vi "project_subject.vi"() -> ()   [LabVIEW 2015]
uses:
  <vilib>/LabVIEW Open Source Project/MQTT Control Packets/Control Packets/SUBACK/Subscription Success Code.ctl
  <vilib>/LabVIEW Open Source Project/MQTT Control Packets/Control Packets/ControlPacket/QualityOfService -- enum.ctl
  <vilib>/LabVIEW Open Source Project/MQTT Control Packets/Control Packets/SUBSCRIBE/Topic Subscription -- cluster.ctl
  <vilib>/LabVIEW Open Source Project/MQTT Control Packets/Control Packets/CONNECT/ConnectFlags -- cluster.ctl
  <vilib>/LabVIEW Open Source Project/MQTT Client/Client class/Client.lvclass/Client.ctl
  <vilib>/LabVIEW Open Source Project/MQTT Connection/MQTT_Base/Base Class/MQTT_Base.lvclass/MQTT_Base.ctl
  <vilib>/LabVIEW Open Source Project/MQTT Control Packets/Control Packets/ControlPacket/ControlPacket.lvclass/ControlPacket.ctl
  <vilib>/Modbus/master/Create Master Instance (Serial).vi
  <vilib>/LabVIEW Open Source Project/MQTT Control Packets/Control Packets/PUBLISH/PUBLISH.lvclass
  <vilib>/Modbus/master/Modbus Master.lvclass
  <vilib>/LabVIEW Open Source Project/MQTT Client/Client class/Client.lvclass
  <vilib>/LabVIEW Open Source Project/MQTT Connection/MQTT_Base/Base Class/MQTT_Base.lvclass
  <vilib>/LabVIEW Open Source Project/MQTT Control Packets/Control Packets/ControlPacket/ControlPacket.lvclass
  <vilib>/LabVIEW Open Source Project/Connection/Connection.TCP/Connection.TCP.lvclass
  <vilib>/LabVIEW Open Source Project/Connection/Connection.LocalQueue/Connection.LocalQueue.lvclass
  <vilib>/LabVIEW Open Source Project/Connection/Connection/Connection.lvclass
  <vilib>/LabVIEW Open Source Project/MQTT Control Packets/Control Packets/SUBACK/SUBACK.lvclass
  <vilib>/LabVIEW Open Source Project/MQTT Control Packets/Control Packets/SUBSCRIBE/SUBSCRIBE.lvclass
  <vilib>/LabVIEW Open Source Project/MQTT Control Packets/Control Packets/CONNECT/CONNECT.lvclass
panel:
  out "source 2":string
  out "code":i32
  out "status":bool
  out "source":string
  in  "stop 2":bool
  out "concatenated string":string
  in  "error in (no error)":errorcluster
  in  "ID (empty:generate new)":string="3822e249-e744-453b-bbf7-de2d9c82744f"
  in  "Connect Flags":T1={"Reserved"=FALSE, "Clean Session"=TRUE, "Will Flag"=FALSE, "Will QoS 1"=FALSE, "Will QoS 2"=FALSE, "Will Retain"=FALSE, "Password Flag"=TRUE, "User Name Flag"=TRUE}
  out "error out 7":errorcluster
  in  "Payload":T2={"Will Topic"="", "Will Message"="", "Username"="FqAEnQLp1Sw4eE9xSTHCFsPptqUtCBk6", "Password"="ruWF9yMR2DR78Q5ppRGFwd8ujJNSitBF"}
  out "error out 2":errorcluster
  out "Incoming Message":u8[](array[numeric]) format="%08b"
  out "error out 6":errorcluster
  out "Data2":string
  out "Type 2":variant
  out "Topic 2":string
  out "error out 5":cluster{}
  out "error out 4":errorcluster
  out "Data1":string
  out "Type":variant
  out "Topic":string
  out "error out 3":cluster{"status":bool, "code":i32}
  in  "Subscribe":bool
  in  "Topic Subscriptions":T3[](array[typedef])=[{"Topic Filter"="@msg/D1/LED1", "QoS"=enum."0 (At Most Once)"}]
  out "Subscription Success":T5[](array[typedef])
  out "Suback":bool
  out "Published":bool
  out "number (0 to 1)":dbl
  in  "Publish":bool
  in  "Stop Client":bool
  in  "SET POINT":dbl
  out "Huminity":dbl(knob) scale=0.0..100.0
  out "Numeric":i32
  out "element":u16
  out "Gauge":dbl(knob) scale=0.0..500.0
  in  "Knob Set Speed":i32(knob) scale=0.0..100.0
  in  "address":u16=100
  in  "holding register value":u16
  in  "Write Button":bool
  in  "baud rate (9600)":u32=9600
  in  "flow control (None)":u16(ring) items=["None", "XON/XOFF", "RTS/CTS", "XON/XOFF & RTS/CTS", "DTR/DSR", "XON/XOFF & DTR/DSR"]
  in  "parity (Even)":u16(ring) items=["None", "Odd", "Even"]
  in  "unit ID":u8=10
  out "error out":errorcluster
  out "register values":u16[](array[numeric])
  in  "number of input registers":u16=10
  in  "starting address":u16=100
  in  "stop":bool
  in  "serial type":enum16{"RTU", "ASCII"}(ring)
  in  "VISA resource name":refnum<visa-resource-name>
  # "The light turns on when the water is turned on."
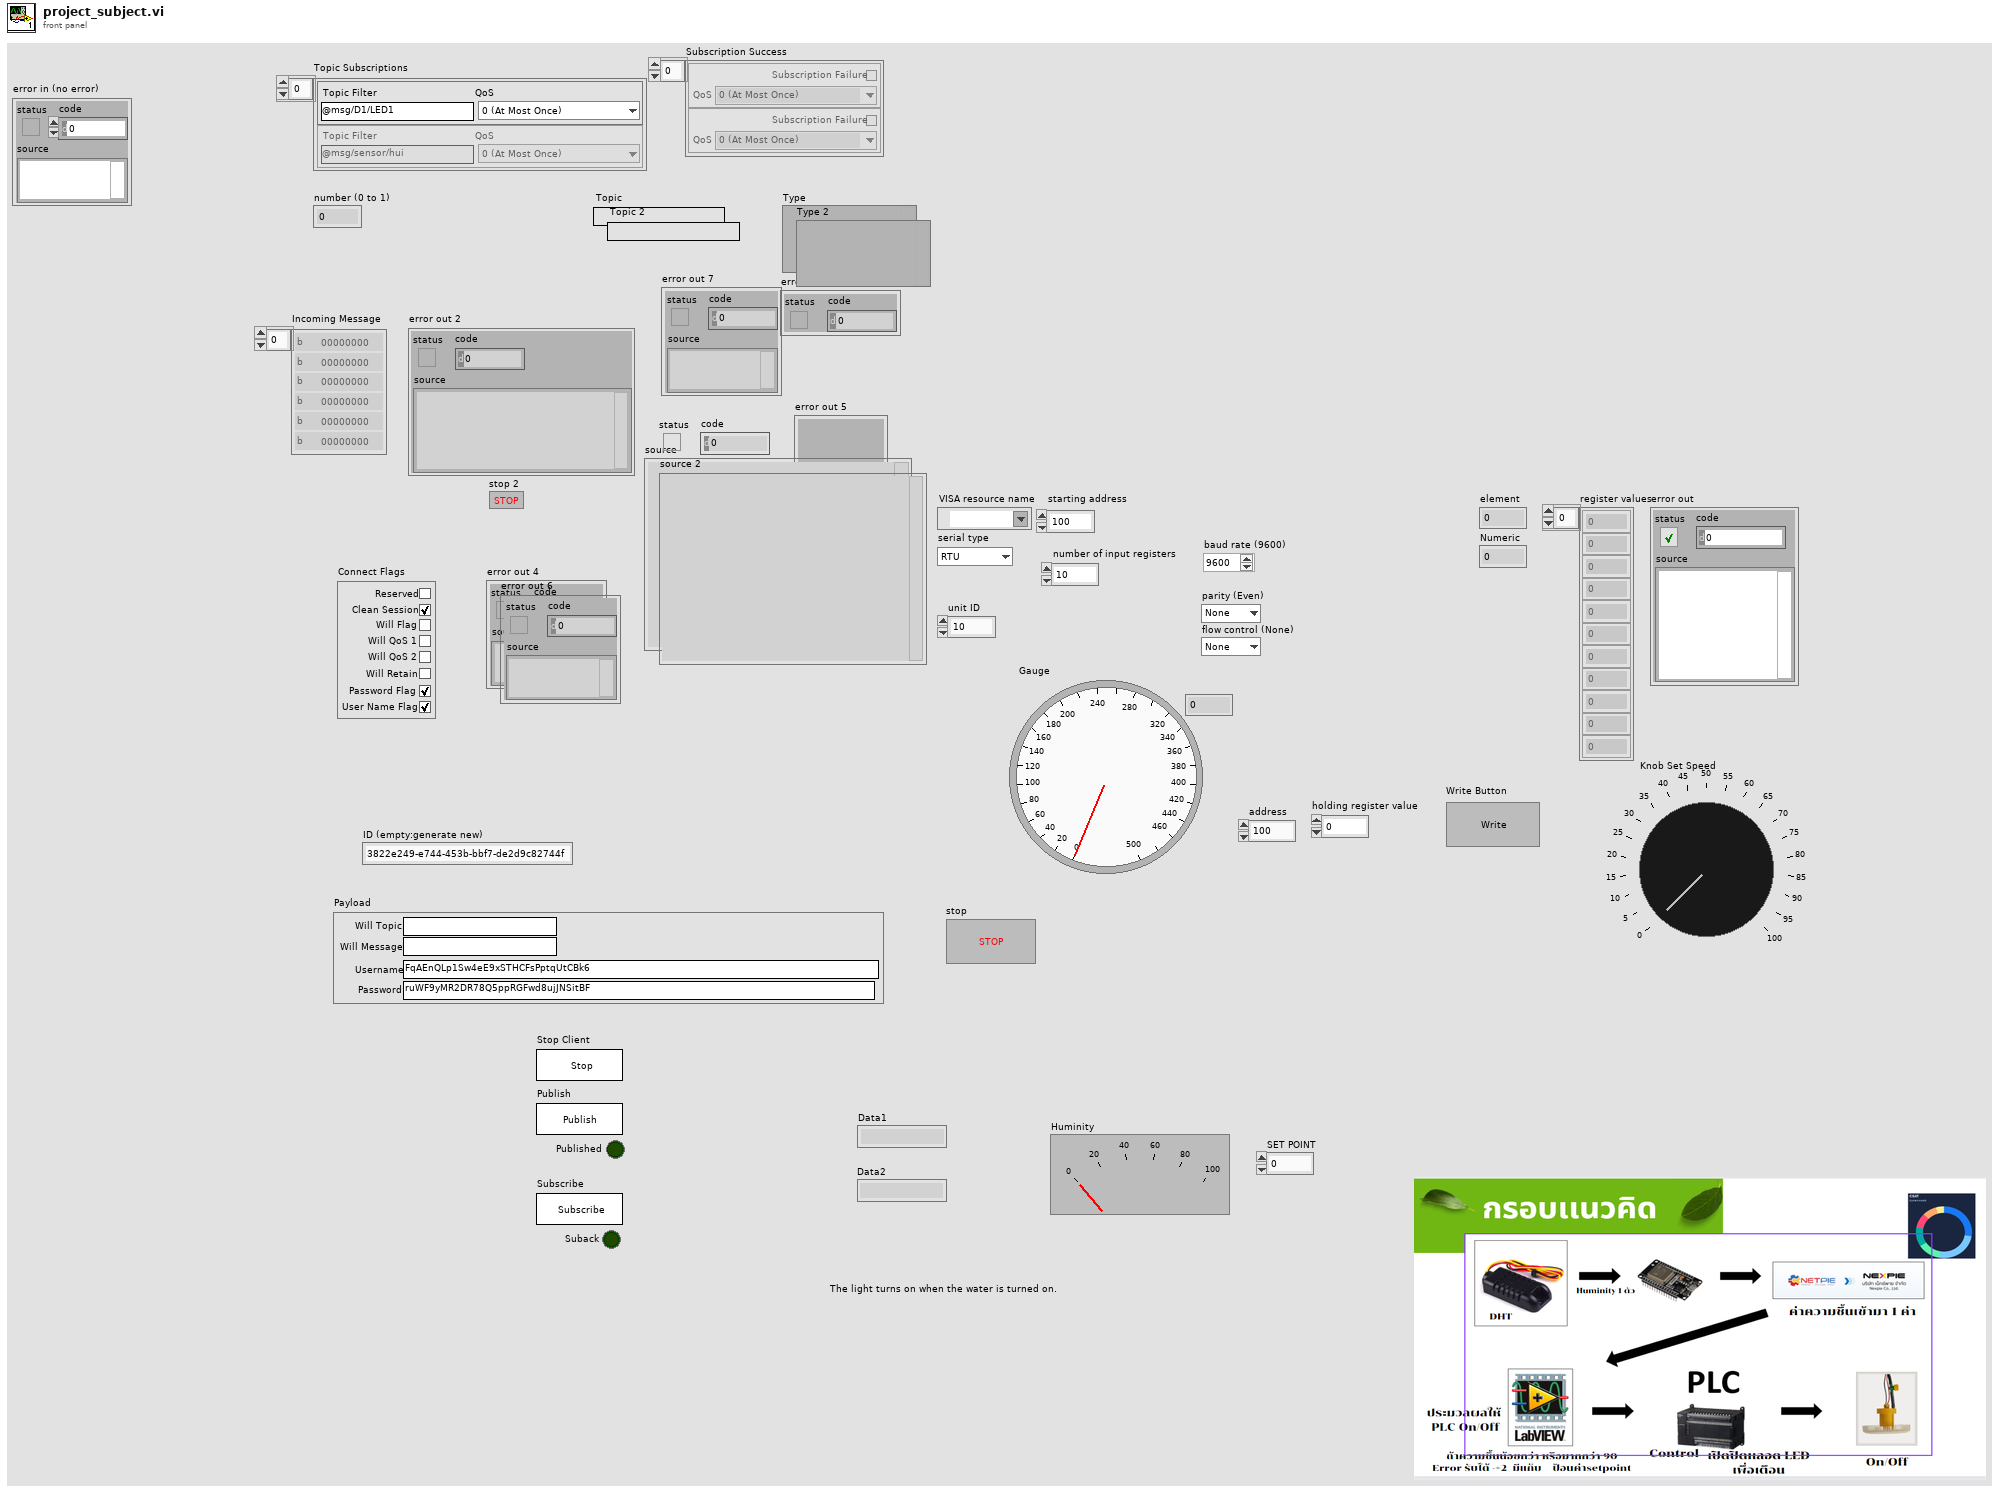
[diagram p1: front panel]
types:
  T1 = typedef "MQTT_Control_Packets.lvlib/CONNECT.lvclass/ConnectFlags -- cluster.ctl" = cluster{"Reserved":bool, "Clean Session":bool, "Will Flag":bool, "Will QoS 1":bool, "Will QoS 2":bool, "Will Retain":bool, "Password Flag":bool, "User Name Flag":bool}
  T2 = cluster{"Will Topic":string, "Will Message":string, "Username":string, "Password":string}
  T3 = typedef "MQTT_Control_Packets.lvlib/SUBSCRIBE.lvclass/Topic Subscription -- cluster.ctl" = cluster{"Topic Filter":string, "QoS":T4}
  T4 = typedef "MQTT_Control_Packets.lvlib/ControlPacket.lvclass/QualityOfService -- enum.ctl" = enum16{"0 (At Most Once)", "1 (At Least Once)", "2 (Exactly Once)"}
  T5 = typedef "MQTT_Control_Packets.lvlib/SUBACK.lvclass/Subscription Success Code.ctl" = cluster{"Subscription Failure":bool, "QoS":T4}
  T6 = typedef "MQTT Client.lvlib/Client.lvclass/Public Events -- cluster.ctl" = cluster{"Connection Status":refnum<user-event>, "Connected":refnum<user-event>, "Application Message":refnum<user-event>}
  T7 = typedef "MQTT Base.lvlib/MQTT_Base.lvclass/Public Events -- cluster.ctl" = cluster{"Stop Event":refnum<user-event>, "Error Event":refnum<user-event>, "Inbound Message":refnum<user-event>}
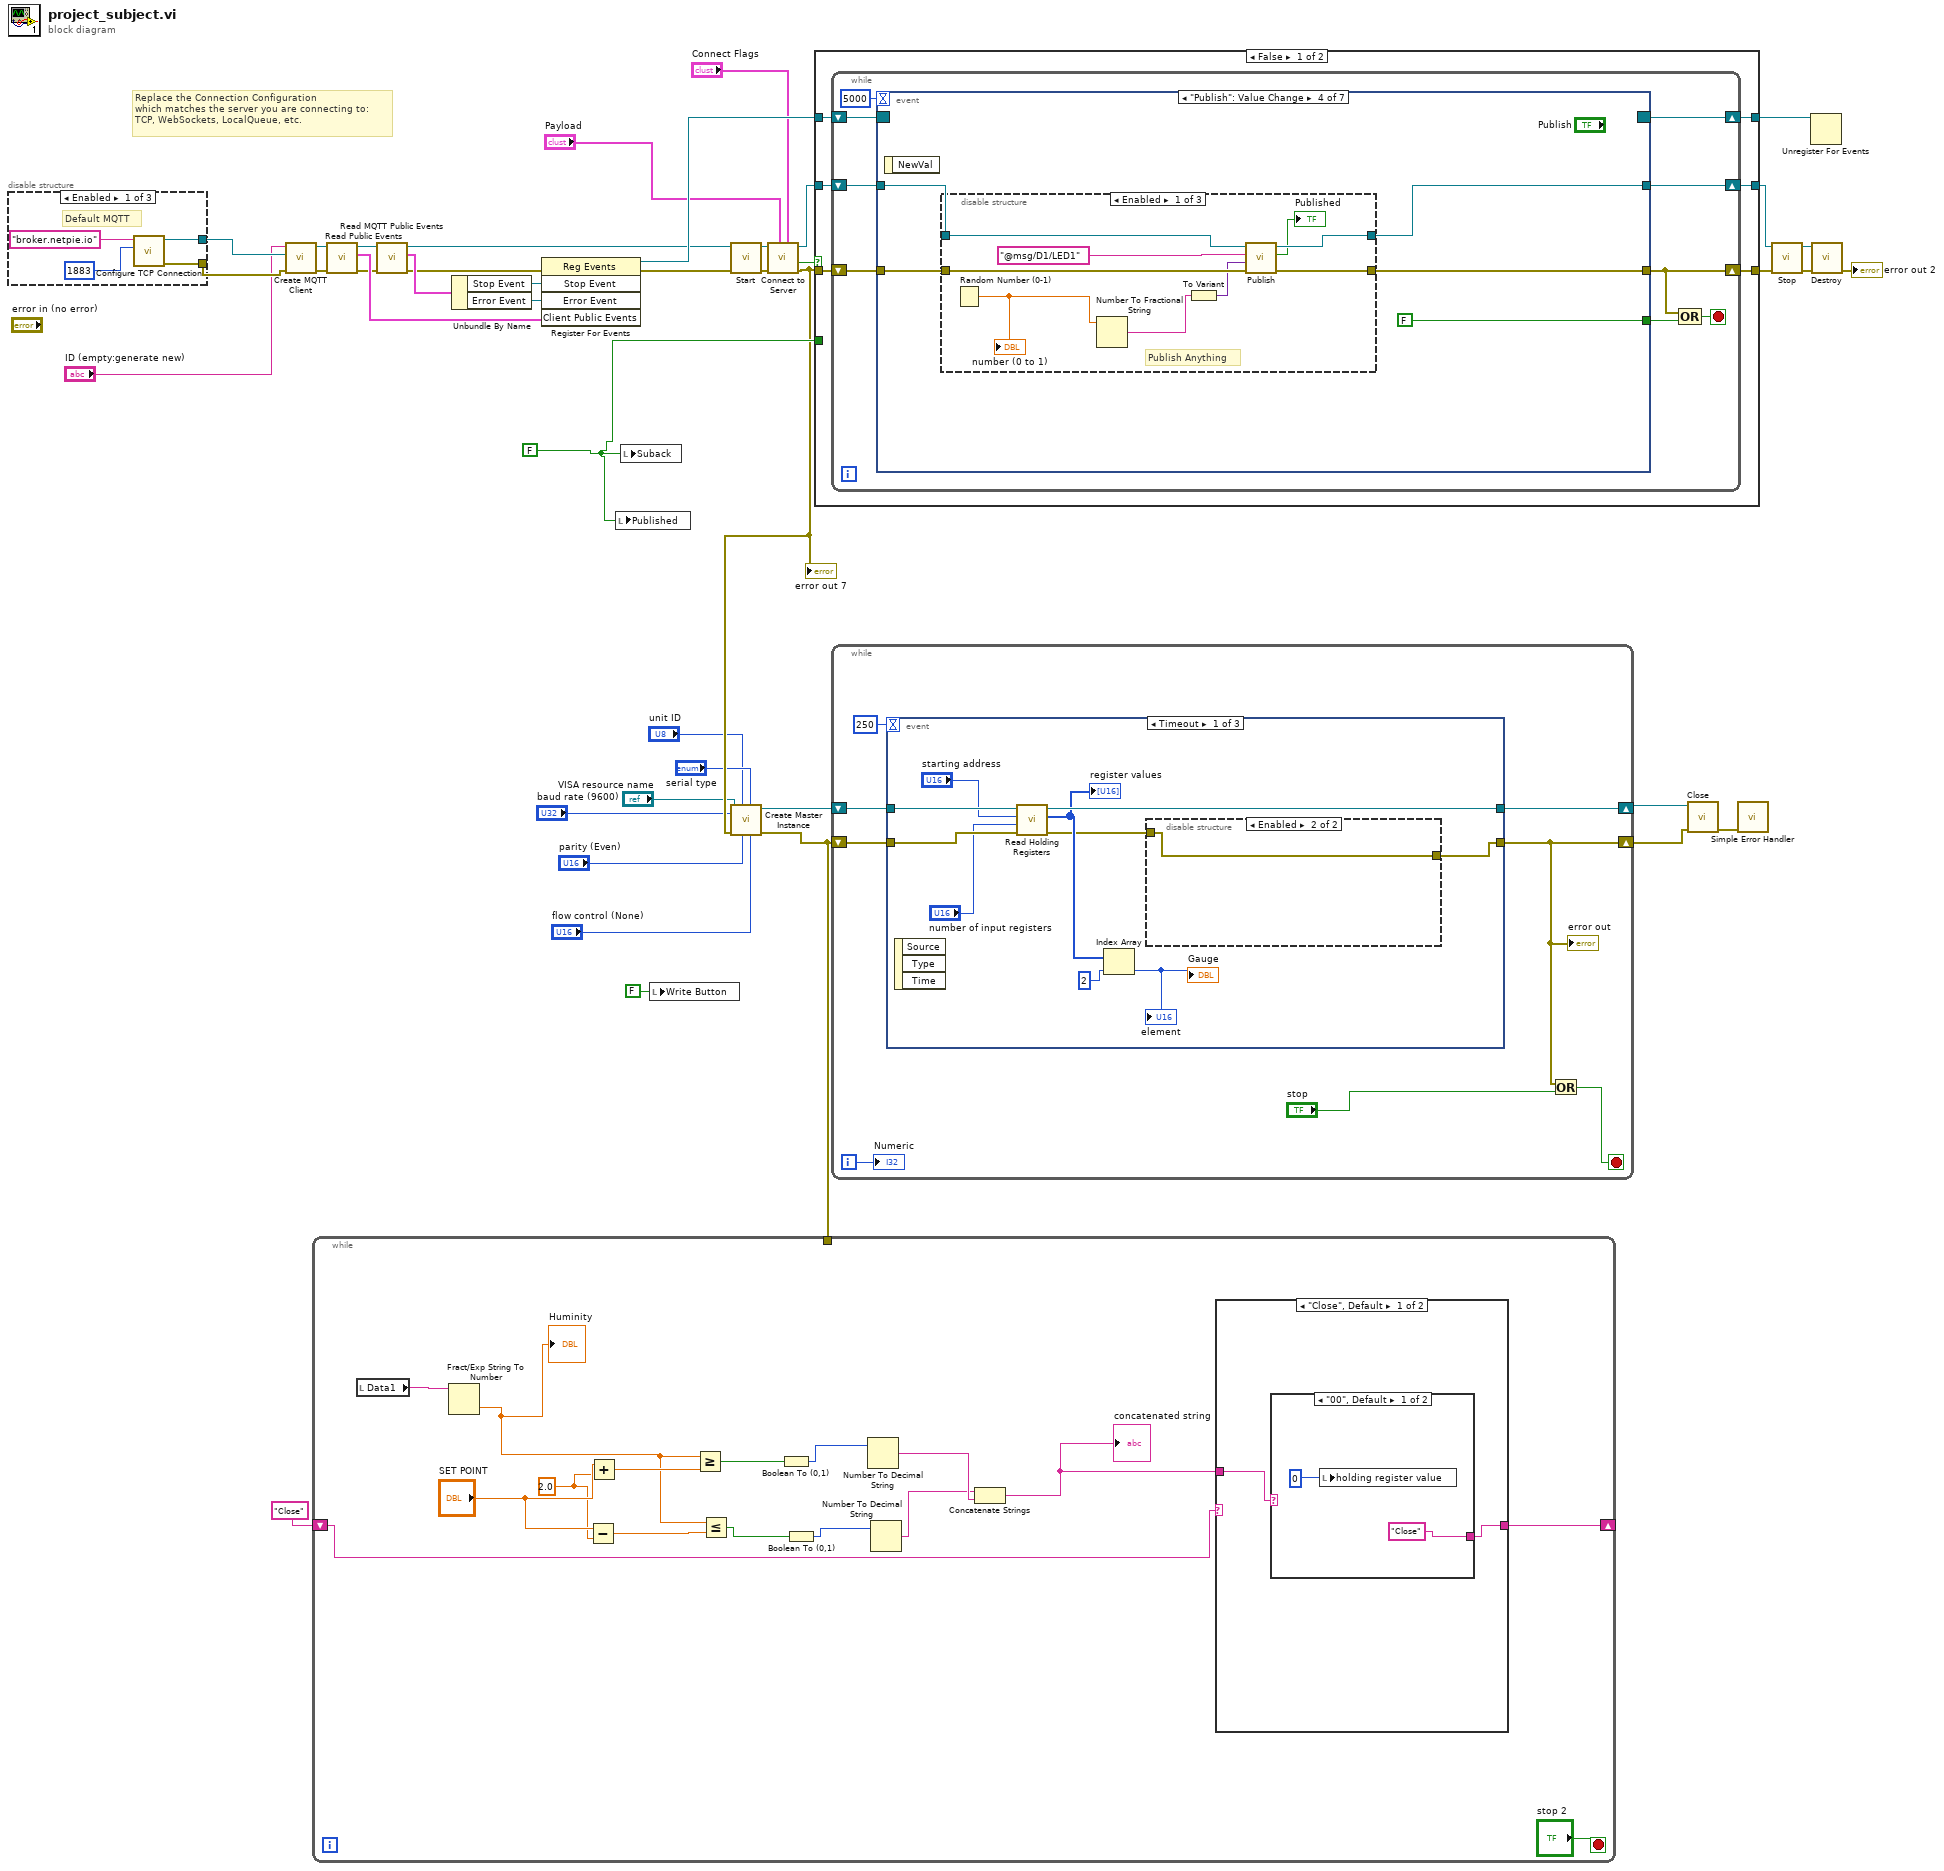
[diagram p0: block diagram]
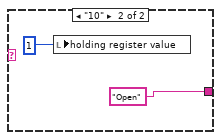
[diagram p2: hidden frame]
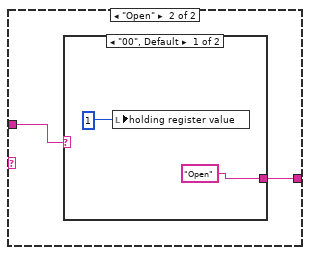
[diagram p3: hidden frame]
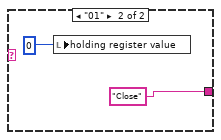
[diagram p4: hidden frame]
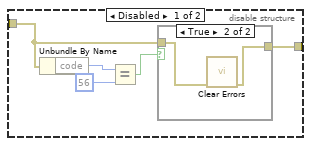
[diagram p5: hidden frame]
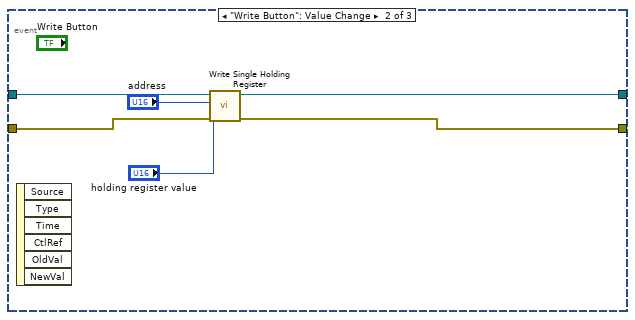
[diagram p7: hidden frame]
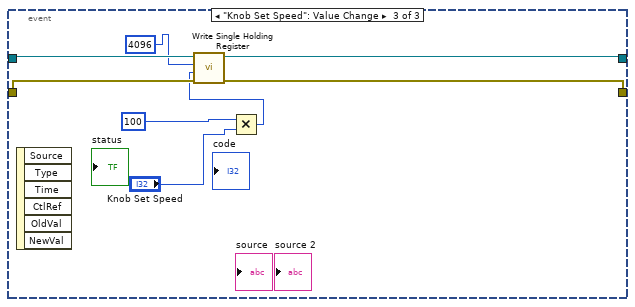
[diagram p8: hidden frame]
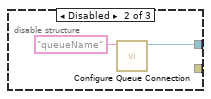
[diagram p9: hidden frame]
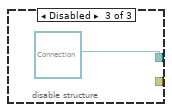
[diagram p10: hidden frame]
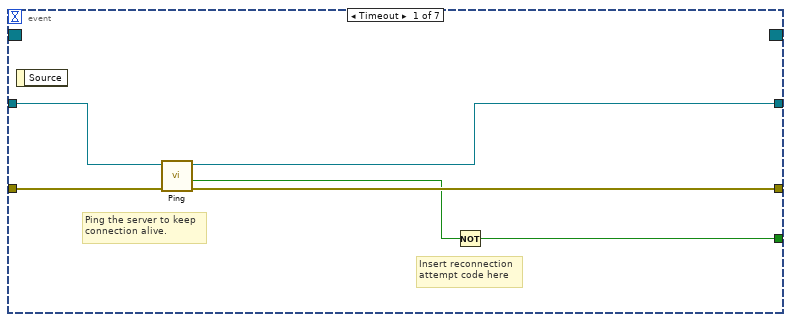
[diagram p11: hidden frame]
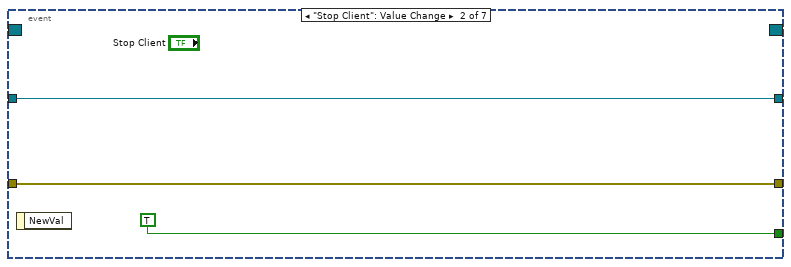
[diagram p12: hidden frame]
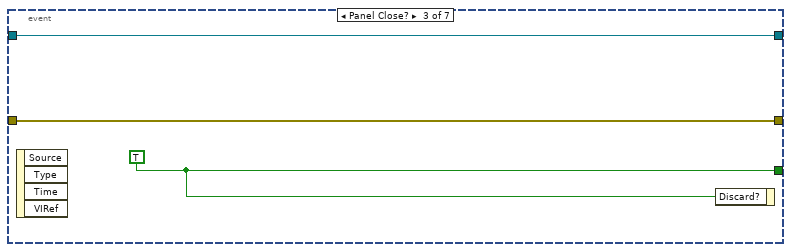
[diagram p13: hidden frame]
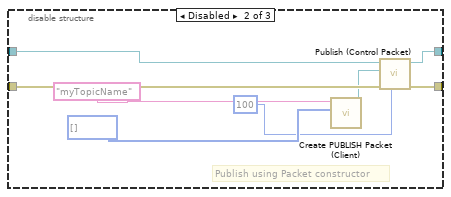
[diagram p14: hidden frame]
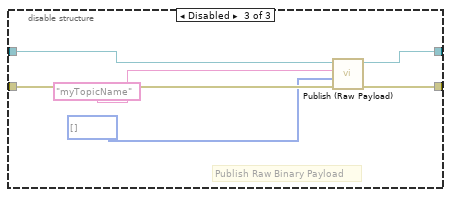
[diagram p15: hidden frame]
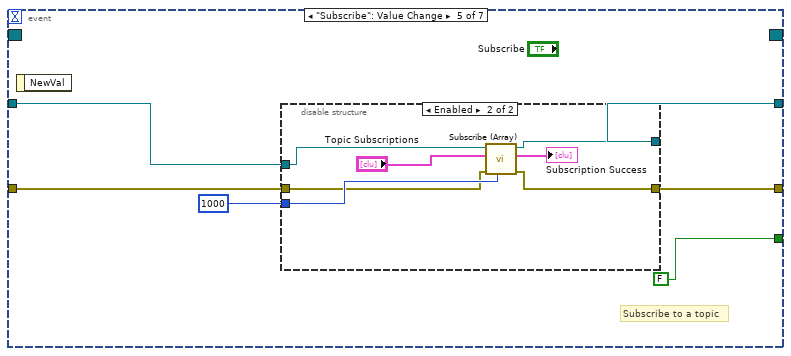
[diagram p16: hidden frame]
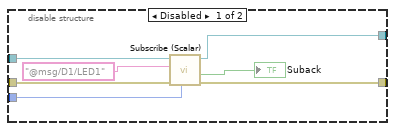
[diagram p17: hidden frame]
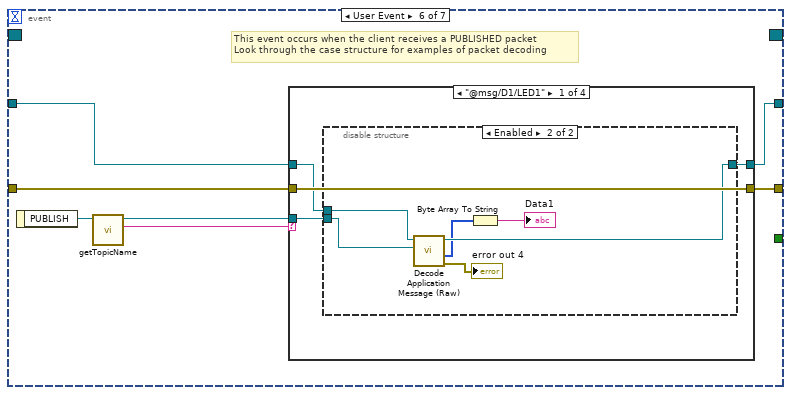
[diagram p18: hidden frame]
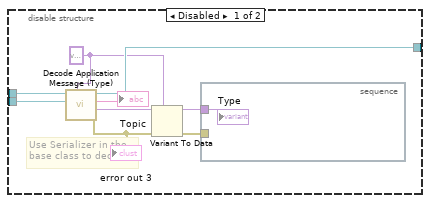
[diagram p19: hidden frame]
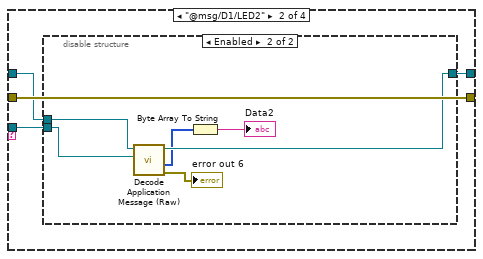
[diagram p20: hidden frame]
diagram:
  w16 = FALSE ("Suback")
  # "Replace the Connection Configuration\nwhich matches the server you are connecting to:\nTCP, WebSockets, LocalQueue, etc."
  n1 = disable-structure shown="Enabled" {
    disable-tunnel: [w45 w48 refnum<class "Connection.lvclass"> refnum ("Connection Configuration")] -> w42
    disable-tunnel: [w43 _ _] -> w19
    frame Enabled {
      # "Default MQTT"
      n2 = call <vilib>:"Configure TCP Connection.vi"("remote port (80)"=u16 1883, "address (localhost)"="broker.netpie.io") -> ("error out"=w43:errorcluster, "Connection.TCP"=w45:refnum<class "Connection.TCP.lvclass">)  [unwired: 8 in]
    }
    frame Disabled {
      n3 = call <vilib>:"Configure Queue Connection.vi"("Queue Name"="queueName") -> ("Connection.LocalQueue"=w48:refnum<class "Connection.LocalQueue.lvclass">)  [unwired: 9 in, 1 out]
    }
    frame Disabled {
    }
  }
  n4 = call <vilib>:"Create MQTT Client.vi"("error in (no error)"=w19, "Connection Configuration"=w42, "ID (empty:generate new)"="ID (empty:generate new)") -> ("error out"=w22:errorcluster, "Client out"=w20:refnum<class "Client.lvclass">)  [unwired: 7 in]
  n5 = call <vilib>:"Read Public Events.vi"("error in (no error)"=w22, "Client in"=w20) -> ("error out"=w23:errorcluster, "Client Public Events"=w25:T6, "Client out"=w21:refnum<class "Client.lvclass">)  [unwired: 7 in]
  n6 = call <vilib>:"Read MQTT Public Events.vi"("error in (no error)"=w23, "MQTT_Base in"=w21) -> ("error out"=w24:errorcluster, "MQTT Public Events"=w36:T7, "MQTT_Base out"=w27:refnum<class "Client.lvclass">)  [unwired: 7 in]
  n7 = Unbundle By Name(w36) -> ("Stop Event"=w34:refnum<user-event>, "Error Event"=w35:refnum<user-event>)
  n8 = register-events(error in=w24, w34, w35, w25) -> (reference out=w30:refnum<event-registration>, error out=w26:errorcluster)  [unwired: 1 in]
  n9 = local write "Published"(w16) -> ()
  n10 = local write "Suback"(w16) -> ()
  n11 = local write "Write Button"(FALSE ("Write Button")) -> ()
  n12 = call <vilib>:"Start.vi"("error in (no error)"=w26, "MQTT_Base in"=w27) -> ("error out"=w29:errorcluster, "MQTT_Base out"=w28:refnum<class "Client.lvclass">)  [unwired: 7 in, 1 out]
  n13 = call <vilib>:"Connect to Server.vi"("Connect Flags"="Connect Flags", "Payload"="Payload", "error in (no error)"=w29, "Client in"=w28) -> ("error out"=w15:errorcluster, "timed out"=w32:bool, "Client out"=w33:refnum<class "Client.lvclass">)  [unwired: 4 in, 1 out]
  "error out 7" <- w15
  n14 = call-poly <vilib>:"Create Master Instance.vi"("flow control (None)"="flow control (None)", "serial type"="serial type", "parity (Even)"="parity (Even)", "unit ID"="unit ID", "error in (no error)"=w15, "baud rate (9600)"="baud rate (9600)", "VISA resource name"="VISA resource name") -> ("error out"=w2:errorcluster, "serial master instance"=w11:refnum<class "Modbus Master.lvclass">)  [unwired: 3 in]
  n15 = while {
    tunnel: w2 -> [_]
    shift-right: [w52] -> _
    shift-left: "Close" -> [w53]
    stop <- "stop 2" stop-if-true
    w63 = 2.0 ("y")
    n16 = local read "Data1"() -> (w65:string)
    n17 = Fract/Exp String To Number(string=w65) -> (number=w50:dbl)  [unwired: 3 in, 1 out]
    "Huminity" <- w50
    n18 = Subtract(x="SET POINT", y=w63) -> (x-y=w61:dbl)
    n19 = Add(x="SET POINT", y=w63) -> (x+y=w62:dbl)
    n20 = Greater Or Equal?(x=w50, y=w62) -> (x >= y?=w60:bool)
    n21 = Less Or Equal?(x=w50, y=w61) -> (x <= y?=w59:bool)
    n22 = Boolean To (0,1)(Boolean=w60) -> (0, 1=w58:i16)
    n23 = Boolean To (0,1)(Boolean=w59) -> (0, 1=w57:i16)
    n24 = Number To Decimal String(number=w58) -> (decimal integer string=w56:string)  [unwired: 1 in]
    n25 = Number To Decimal String(number=w57) -> (decimal integer string=w55:string)  [unwired: 1 in]
    n26 = Concatenate Strings(w55, w56) -> (w54:string)
    "concatenated string" <- w54
    n27 = case shown="\"Close\", Default" w53 {
      tunnel: w54 -> [w66 w73]
      tunnel: [w67 w72] -> w52
      frame "Close", Default {
        n28 = case shown="\"00\", Default" w66 {
          tunnel: ["Close" "Open"] -> w67
          frame "00", Default {
            n29 = local write "holding register value"(u16 0 ("holding register value")) -> ()
          }
          frame "10" {
            n30 = local write "holding register value"(u16 1 ("holding register value")) -> ()
          }
        }
      }
      frame "Open" {
        n31 = case shown="\"00\", Default" w73 {
          tunnel: ["Open" "Close"] -> w72
          frame "00", Default {
            n32 = local write "holding register value"(u16 1 ("holding register value")) -> ()
          }
          frame "01" {
            n33 = local write "holding register value"(u16 0 ("holding register value")) -> ()
          }
        }
      }
    }
  }
  n34 = case shown="False" w32 {
    tunnel: w30 -> [w83 w215]
    tunnel: [w82 w215] -> w31
    tunnel: w15 -> [w79 w213]
    tunnel: w33 -> [w81 w214]
    tunnel: [w80 w214] -> w38
    tunnel: [w78 w213] -> w40
    tunnel: w16 -> [_ _]
    frame False {
      n35 = while {
        shift-right: [w91] -> w82
        shift-left: w83 -> [w92]
        shift-right: [w84] -> w80
        shift-left: w81 -> [w85]
        shift-right: [w89] -> w78
        shift-left: w79 -> [w90]
        stop <- w88 stop-if-true
        n36 = event shown="[3] \"Publish\": Value Change" {
          selector: w92 -> [_ _ _ _ _ _ _]
          dyn-events: [_ _ _ _ _ _ _] -> w91
          timeout: 5000 -> [_ _ _ _ _ _ _]
          tunnel: w90 -> [w97 w100 w102 w107 w136 w154 w212]
          tunnel: [w95 w100 w102 w106 w135 w155 w212] -> w89
          tunnel: [w94 TRUE w104 FALSE FALSE _ TRUE] -> w87
          tunnel: w85 -> [w98 w101 w103 w108 w137 w157 w210]
          tunnel: [w96 w101 w103 w105 w134 w156 w210] -> w84
          event Timeout {
            # "Insert reconnection\nattempt code here"
            # "Ping the server to keep\nconnection alive."
            n37 = event-data() -> ()  [unwired: 1 in, 1 out]
            n38 = call <vilib>:"Ping.vi"("error in (no error)"=w97, "Client in"=w98) -> ("error out"=w95:errorcluster, "Server responded"=w93:bool, "Client out"=w96:refnum<class "Client.lvclass">)  [unwired: 6 in, 1 out]
            n39 = Not(x=w93) -> (.not. x?=w94:bool)
          }
          event "Stop Client": Value Change {
            n40 = event-data() -> ()  [unwired: 1 in, 1 out]
          }
          event Panel Close? {
            w104 = TRUE
            n41 = event-data() -> ()  [unwired: 1 in, 4 out]
            n42 = event-data("Discard?"=w104) -> ()  [unwired: 1 in, 1 out]
          }
          event "Publish": Value Change {
            n43 = event-data() -> ()  [unwired: 1 in, 1 out]
            n44 = disable-structure shown="Enabled" {
              disable-tunnel: w108 -> [w118 w124 w132]
              disable-tunnel: w107 -> [w117 w122 w129]
              disable-tunnel: [w116 w121 w130] -> w106
              disable-tunnel: [w115 w123 w131] -> w105
              frame Enabled {
                # "Publish Anything"
                n45 = Random Number (0-1)() -> (number: 0 to 1=w111:dbl)
                "number (0 to 1)" <- w111
                n46 = Number To Fractional String(number=w111) -> (F-format string=w110:string)  [unwired: 3 in]
                n47 = To Variant(anything=w110) -> (Variant=w113:variant)
                n48 = call <vilib>:"Publish.vi"("error in (no error)"=w117, "Payload"=w113, "Topic Name (empty: Payload name)"="@msg/D1/LED1", "Client in"=w118) -> ("error out"=w116:errorcluster, "Published"=→"Published":bool, "Client out"=w115:refnum<class "Client.lvclass">)  [unwired: 5 in]
              }
              frame Disabled {
                # "Publish using Packet constructor"
                n49 = call <vilib>:"Create PUBLISH Packet (Client).vi"("Payload"=u8[] [], "Topic Name"="myTopicName" ("Topic Name (empty: Payload name)")) -> ("PUBLISH"=w119:refnum<class "PUBLISH.lvclass">)  [unwired: 6 in, 3 out]
                n50 = call <vilib>:"Publish (Control Packet).vi"("timeout (1000ms)"=100 ("timeout (0ms : no ack)"), "error in (no error)"=w122, "PUBLISH"=w119, "Client in"=w124) -> ("error out"=w121:errorcluster, "Client out"=w123:refnum<class "Client.lvclass">)  [unwired: 5 in, 1 out]
              }
              frame Disabled {
                # "Publish Raw Binary Payload"
                n51 = call <vilib>:"Publish (Raw Payload).vi"("error in (no error)"=w129, "Binary Payload"=u8[] [] ("Payload"), "Topic Name"="myTopicName" ("Topic Name (empty: Payload name)"), "Client in"=w132) -> ("error out"=w130:errorcluster, "Client out"=w131:refnum<class "Client.lvclass">)  [unwired: 5 in, 1 out]
              }
            }
          }
          event "Subscribe": Value Change {
            # "Subscribe to a topic"
            n52 = event-data() -> ()  [unwired: 1 in, 1 out]
            n53 = disable-structure shown="Enabled" {
              disable-tunnel: w137 -> [w145 w152]
              disable-tunnel: w136 -> [w143 w148]
              disable-tunnel: [w142 w147] -> w135
              disable-tunnel: [w141 w149] -> w134
              disable-tunnel: 1000 ("timeout (100ms)") -> [w139 w151]
              frame Disabled {
                n54 = call <vilib>:"Subscribe (Scalar).vi"("timeout (1000ms)"=w139, "error in (no error)"=w143, "Topic Filter"="@msg/D1/LED1" ("Topic Name (empty: Payload name)"), "Client in"=w145) -> ("error out"=w142:errorcluster, "Ack"=→"Suback":bool, "Client out"=w141:refnum<class "Client.lvclass">)  [unwired: 5 in]
              }
              frame Enabled {
                n55 = call <vilib>:"Subscribe (Array).vi"("timeout (1000ms)"=w151, "error in (no error)"=w148, "Topic Subscriptions"="Topic Subscriptions", "Client in"=w152) -> ("error out"=w147:errorcluster, "Subscription Success"=→"Subscription Success":T5[], "Client out"=w149:refnum<class "Client.lvclass">)  [unwired: 5 in]
              }
            }
          }
          event User Event {
            # "This event occurs when the client receives a PUBLISHED packet\nLook through the case structure for examples of packet decoding"
            n56 = event-data() -> ("PUBLISH"=w159:refnum<class "PUBLISH.lvclass">)  [unwired: 1 in]
            n57 = call <vilib>:"getTopicName.vi"("PUBLISH in"=w159) -> ("Topic"=w158:string, "PUBLISH out"=w153:refnum<class "PUBLISH.lvclass">)  [unwired: 8 in, 1 out]
            n58 = case shown="\"@msg/D1/LED1\"" w158 {
              tunnel: w157 -> [w162 w182 w205 w209]
              tunnel: [w161 w181 w204 w209] -> w156
              tunnel: [w163 w183 w202 w208] -> w155
              tunnel: w154 -> [w163 w183 w201 w208]
              tunnel: w153 -> [w160 w180 w200 w207]
              frame "@msg/D1/LED1" {
                n59 = disable-structure shown="Enabled" {
                  disable-tunnel: w162 -> [w170 w179]
                  disable-tunnel: [w169 w177] -> w161
                  disable-tunnel: w160 -> [w168 w178]
                  frame Disabled {
                    w166 = variant ("Type")
                    # "Use Serializer in the\nbase class to decode"
                    n60 = call <vilib>:"Decode Application Message (Type).vi"("Type"=w166, "PUBLISH"=w168, "Client in"=w170) -> ("error out"=w165:errorcluster, "Payload"=w167:variant, "Topic"=→"Topic":string, "Client out"=w169:refnum<class "Client.lvclass">)  [unwired: 5 in]
                    "error out 3" <- w165
                    n61 = Variant To Data(error in=w165, type=w166, Variant=w167) -> (data=w172:variant, error out=w171:errorcluster)
                    n62 = stacked-sequence {
                      tunnel: w172 -> [w173]
                      tunnel: w171 -> [_]
                      frame #0 {
                        "Type" <- w173
                      }
                    }
                  }
                  frame Enabled {
                    n63 = call <vilib>:"Decode Application Message (Raw).vi"("PUBLISH"=w178, "Client in"=w179) -> ("error out"=→"error out 4":errorcluster, "Payload"=w175:u8[], "Client out"=w177:refnum<class "Client.lvclass">)  [unwired: 6 in, 1 out]
                    n64 = Byte Array To String(unsigned byte array=w175) -> (string=→"Data1":string)
                  }
                }
              }
              frame "@msg/D1/LED2" {
                n65 = disable-structure shown="Enabled" {
                  disable-tunnel: w182 -> [w190 w199]
                  disable-tunnel: [w189 w197] -> w181
                  disable-tunnel: w180 -> [w188 w198]
                  frame Disabled {
                    w186 = variant ("Type")
                    # "Use Serializer in the\nbase class to decode"
                    n66 = call <vilib>:"Decode Application Message (Type).vi"("Type"=w186, "PUBLISH"=w188, "Client in"=w190) -> ("error out"=w185:errorcluster, "Payload"=w187:variant, "Topic"=→"Topic 2":string, "Client out"=w189:refnum<class "Client.lvclass">)  [unwired: 5 in]
                    "error out 5" <- w185
                    n67 = Variant To Data(error in=w185, type=w186, Variant=w187) -> (data=w192:variant, error out=w191:errorcluster)
                    n68 = stacked-sequence {
                      tunnel: w192 -> [w193]
                      tunnel: w191 -> [_]
                      frame #0 {
                        "Type 2" <- w193
                      }
                    }
                  }
                  frame Enabled {
                    n69 = call <vilib>:"Decode Application Message (Raw).vi"("PUBLISH"=w198, "Client in"=w199) -> ("error out"=→"error out 6":errorcluster, "Payload"=w195:u8[], "Client out"=w197:refnum<class "Client.lvclass">)  [unwired: 6 in, 1 out]
                    n70 = Byte Array To String(unsigned byte array=w195) -> (string=→"Data2":string)
                  }
                }
              }
              frame "RawPayload" {
                n71 = call <vilib>:"Decode Application Message (Raw).vi"("error in (no error)"=w201, "PUBLISH"=w200, "Client in"=w205) -> ("error out"=w202:errorcluster, "Payload"=w203:u8[], "Client out"=w204:refnum<class "Client.lvclass">)  [unwired: 5 in, 1 out]
                n72 = stacked-sequence {
                  tunnel: w203 -> [_]
                  frame #0 {
                  }
                }
              }
              frame Default {
                # "Read Raw Payload"
                n73 = call <vilib>:"Read Payload.vi"("ControlPacket in"=w207) -> ("Payload"=→"Incoming Message":u8[])  [unwired: 9 in, 1 out]
              }
            }
          }
          event User Event {
            n74 = event-data() -> ()  [unwired: 1 in, 1 out]
          }
        }
        n75 = Compound Arithmetic op=OR(w89, w87) -> (w88:bool)
      }
    }
    frame True {
    }
  }
  n76 = while {
    shift-right: [w220] -> w8
    shift-left: w11 -> [w223]
    shift-right: [w219] -> w9
    shift-left: w2 -> [w222]
    i -> [w216]
    stop <- w221 stop-if-true
    n77 = event shown="[0] Timeout" {
      selector: _ -> [_ _ _]
      dyn-events: _ -> [_ _ _]
      timeout: 250 -> [_ _ _]
      tunnel: w223 -> [w233 w248 w256]
      tunnel: w222 -> [w232 w247 w254]
      tunnel: [w231 w246 w255] -> w220
      tunnel: [w224 w245 w253] -> w219
      event Timeout {
        n78 = event-data() -> ()  [unwired: 1 in, 3 out]
        n79 = call-dynamic "Read Holding Registers.vi"("error in (no error)"=w232, "number of holding registers"="number of input registers", "starting address"="starting address", "Modbus master in"=w233) -> ("error out"=w225:errorcluster, "register values"=w228:u16[], "Modbus master out"=w231:refnum<class "Modbus Master.lvclass">)  [unwired: 5 in]
        "register values" <- w228
        n80 = Index Array(array=w228, index=2) -> (element=→"Gauge" →"element":u16)
        n81 = disable-structure shown="Enabled" {
          disable-tunnel: w225 -> [w235 w242]
          disable-tunnel: [w234 w242] -> w224
          frame Disabled {
            n82 = Unbundle By Name(w235) -> ("code"=w238:i32)
            n83 = Equal?(x=w238, y=56) -> (x = y?=w236:bool)
            n84 = case shown="True" w236 {
              tunnel: w235 -> [w239 w241]
              tunnel: [w239 w240] -> w234
              frame False {
              }
              frame True {
                n85 = call <vilib>:"Clear Errors.vi"("error in (no error)"=w241) -> ("error out"=w240:errorcluster)  [unwired: 5 in, 1 out]
              }
            }
          }
          frame Enabled {
          }
        }
      }
      event "Write Button": Value Change {
        n86 = event-data() -> ()  [unwired: 1 in, 6 out]
        n87 = call-dynamic "Write Single Holding Register.vi"("error in (no error)"=w247, "holding register value"="holding register value", "address"="address", "Modbus master in"=w248) -> ("error out"=w245:errorcluster, "Modbus master out"=w246:refnum<class "Modbus Master.lvclass">)  [unwired: 6 in]
      }
      event "Knob Set Speed": Value Change {
        n88 = event-data() -> ()  [unwired: 1 in, 6 out]
        n89 = Multiply(x=100, y="Knob Set Speed") -> (x*y=w250:i32)
        n90 = call-dynamic "Write Single Holding Register.vi"("error in (no error)"=w254, "holding register value"=w250, "address"=u16 4096, "Modbus master in"=w256) -> ("error out"=w253:errorcluster, "Modbus master out"=w255:refnum<class "Modbus Master.lvclass">)  [unwired: 6 in]
      }
    }
    "error out" <- w219
    n91 = Or(x=w219, y="stop") -> (x .or. y?=w221:bool)
    "Numeric" <- w216
  }
  n92 = call-dynamic "Close.vi"("error in (no error)"=w9, "Modbus master in"=w8) -> ("error out"=w7:errorcluster)  [unwired: 9 in]
  n93 = call <vilib>:"Simple Error Handler.vi"("error in (no error)"=w7) -> ()  [unwired: 4 in, 5 out]
  n94 = call <vilib>:"Stop.vi"("error in (no error)"=w40, "MQTT_Base in"=w38) -> ("error out"=w39:errorcluster, "MQTT_Base out"=w37:refnum<class "Client.lvclass">)  [unwired: 7 in, 1 out]
  n95 = Unregister For Events(event registration refnum=w31) -> ()  [unwired: 1 in, 1 out]
  n96 = call <vilib>:"Destroy.vi"("error in (no error)"=w39, "MQTT_Base in"=w37) -> ("error out"=→"error out 2":errorcluster)  [unwired: 8 in, 1 out]
